vi "Set flags logic-at acquisition start.vi"(8 "error in (no error)":errorcluster, 9 "Imaging Protocol":T1) -> (0 "error out":errorcluster)   [LabVIEW 2020]
uses:
  Typedefs/Imaging Protocols enum.ctl
  Typedefs/Read Write Enum.ctl
  typedefs/Functions enum.ctl
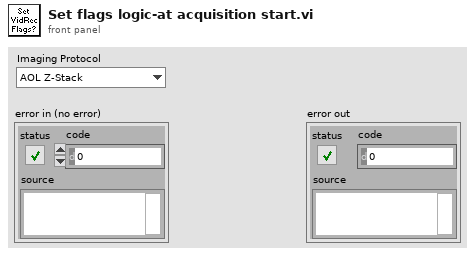
[diagram p1: front panel]
types:
  T1 = typedef "Imaging Protocols enum.ctl" = enum16{"AOL Z-Stack", "Motor Z Stack", "Functional Acquisition", "Single Plane Acquisition", "Volume Acquisition", "Live Imaging", "Live Plane Imaging", "Live Volume Imaging"}
  T2 = typedef "Read Write Enum.ctl" = enum16{"Read", "Write"}
  T3 = typedef "Functions enum.ctl" = enum16{"Create", "Start", "Write", "Stop", "Clear"}
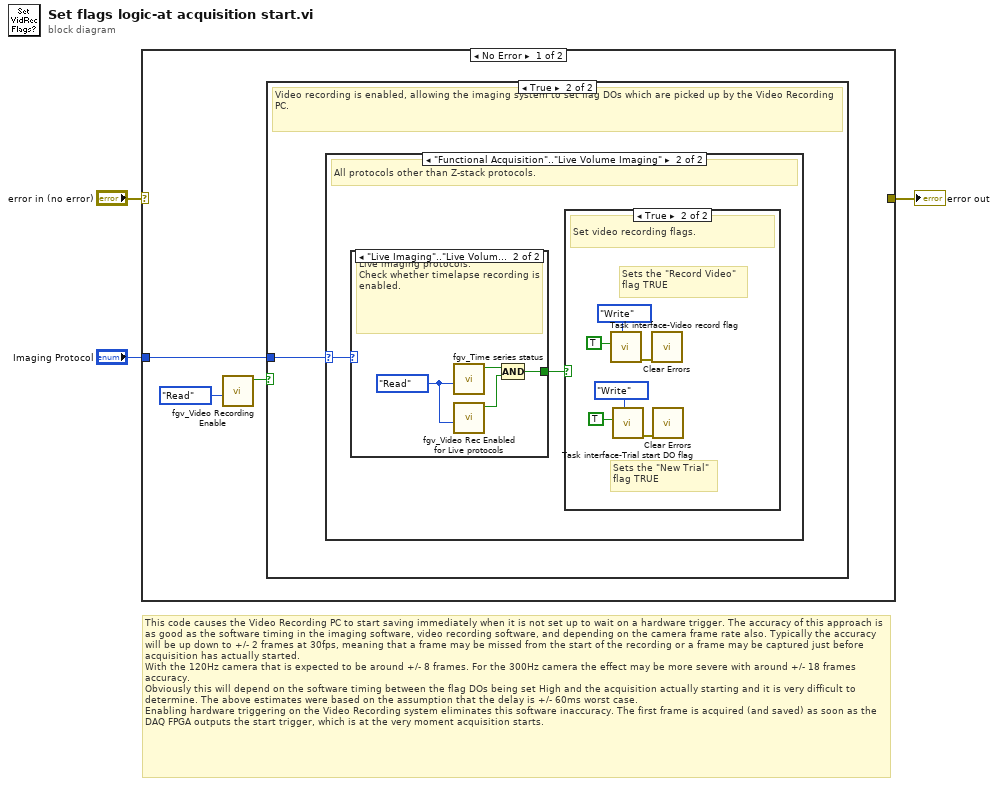
[diagram p0: block diagram]
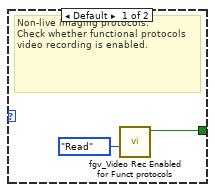
[diagram p5: hidden frame]
diagram:
  # "This code causes the Video Recording PC to start saving immediately when it is not set up to wait on a hardware trigger. The accuracy of this approach is as good as the software timing in the imaging software, video recording software, and depending on the camera frame rate also. Typically the accuracy will be up down to +/- 2 frames at 30fps, meaning that a frame may be missed from the start of the recording or a frame may be captured just before acquisition has actually started.\nWith the 120Hz camera that is expected to be around +/- 8 frames. For the 300Hz camera the effect may be more severe with around +/- 18 frames accuracy.\nObviously this will depend on the software timing between the flag DOs being set High and the acquisition actually starting and it is very difficult to determine. The above estimates were based on the assumption that the delay is +/- 60ms worst case.\nEnabling hardware triggering on the Video Recording system eliminates this software inaccuracy. The first frame is acquired (and saved) as soon as the DAQ FPGA outputs the start trigger, which is at the very moment acquisition starts."
  n1 = case shown="No Error" "error in (no error)" {
    selector: "error in (no error)" -> [_ w22]
    tunnel: [_ w22] -> w2
    tunnel: "Imaging Protocol" -> [w4 _]
    frame No Error {
      n2 = call "fgv_Video Recording Enable.vi"("Function"=Read_Write_Enum."Read") -> ("Video Recording Enabled"=w6:bool)  [unwired: 9 in, 1 out]
      n3 = case shown="True" w6 {
        tunnel: w4 -> [_ w7]
        frame False {
          # "Video recording is disabled. No flag DOs are set. The Video Recording PC will still show live video streams but \nwill not record any videos."
        }
        frame True {
          # "Video recording is enabled, allowing the imaging system to set flag DOs which are picked up by the Video Recording PC."
          n4 = case shown="\"Functional Acquisition\"..\"Live Volume Imaging\"" w7 {
            selector: w7 -> [_ w9]
            frame Default {
              # "Z stack protocols (no video recording ever during such protocols)"
            }
            frame "Functional Acquisition".."Live Volume Imaging" {
              # "All protocols other than Z-stack protocols."
              n5 = case shown="\"Live Imaging\"..\"Live Volume Imaging\"" w9 {
                tunnel: [w16 w19] -> w8
                frame Default {
                  # "Non-live imaging protocols.\nCheck whether functional protocols video recording is enabled."
                  n6 = call "fgv_Video Rec Enabled for Funct protocols.vi"("Function"=Read_Write_Enum."Read") -> ("Video Recording Enabled for functional acq protocols"=w16:bool)  [unwired: 10 in]
                }
                frame "Live Imaging".."Live Volume Imaging" {
                  w18 = Read_Write_Enum."Read" ("Function")
                  # "Live imaging protocols.\nCheck whether timelapse recording is enabled."
                  n7 = call "fgv_Time series status.vi"("Function"=w18) -> ("Timelapse?"=w20:bool)  [unwired: 10 in]
                  n8 = call "fgv_Video Rec Enabled for Live protocols.vi"("Function"=w18) -> ("Video Recording Enabled for Live protocols"=w21:bool)  [unwired: 10 in]
                  n9 = Compound Arithmetic op=AND(w20, w21) -> (w19:bool)
                }
              }
              n10 = case shown="True" w8 {
                frame False {
                  # "Do nothing."
                }
                frame True {
                  # "Sets the \"New Trial\"\nflag TRUE"
                  # "Sets the \"Record Video\"\nflag TRUE"
                  # "Set video recording flags."
                  n11 = call "Task interface-Video record flag.vi"("Function"=Functions_enum."Write", "DO value"=TRUE) -> ("error out"=w14:errorcluster)  [unwired: 9 in]
                  n12 = call "Task interface-Trial start DO flag.vi"("Function"=Functions_enum."Write", "DO value"=TRUE) -> ("error out"=w10:errorcluster)  [unwired: 9 in]
                  n13 = call <vilib>:"Clear Errors.vi"("error in (no error)"=w14) -> ()  [unwired: 5 in, 2 out]
                  n14 = call <vilib>:"Clear Errors.vi"("error in (no error)"=w10) -> ()  [unwired: 5 in, 2 out]
                }
              }
            }
          }
        }
      }
    }
    frame Error {
    }
  }
  "error out" <- w2
